vi "excelrowconcat_singlecol_LR_HR.vi"() -> ()   [LabVIEW 2020]
uses:
  <vilib>/addons/_office/excel.llb/Excel Get Data ([dbl]).vi
  <vilib>/Utility/file.llb/Write To Spreadsheet File (DBL).vi
  <vilib>/Utility/NIReport.llb/NI_report.lvclass
  <vilib>/Utility/NIReport.llb/Excel/NI_Excel.lvclass
  <vilib>/addons/_office/NI_ReportGenerationToolkit.lvlib
panel:
  out "Total LR Selected Row":i32=3
  in  "Tab Control":enum32{"HR", "LR"}(tab)=enum."LR"
  out "HR selected row":ext[](array[numeric])=[5.0, 20.0, 35.0, 50.0] format="%#_6f"
  out "HR Sheet Values":ext[][](array[numeric])=[[1.0, 16.0, 31.0, 46.0], [2.0, 17.0, 32.0, 47.0], [3.0, 18.0, 33.0, 48.0], [4.0, 19.0, 34.0, 49.0], [5.0, 20.0, 35.0, 50.0], [6.0, 21.0, 36.0, 51.0], [7.0, 22.0, 37.0, 52.0], [8.0, 23.0, 38.0, 53.0], [9.0, 24.0, 39.0, 54.0], [10.0, 25.0, 40.0, 55.0], [11.0, 26.0, 41.0, 56.0], [12.0, 27.0, 42.0, 57.0], [13.0, 28.0, 43.0, 58.0], [14.0, 29.0, 44.0, 59.0], [15.0, 30.0, 45.0, 60.0]] format="%_6f"
  out "HR Added row":ext[][](array[numeric])=[[1.0, 16.0, 31.0, 46.0], [3.0, 18.0, 33.0, 48.0], [5.0, 20.0, 35.0, 50.0]] format="%#_6f"
  out "HR Selected Column":ext[](array[numeric])=[46.0, 48.0, 50.0] format="%#_6f"
  out "HR Stack Col":ext[](array[numeric])=[1.0, 3.0, 5.0, 16.0, 18.0, 20.0, 31.0, 33.0, 35.0, 46.0, 48.0, 50.0] format="%#_6f"
  out "Rows":i32=15
  out "Columns":i32=4
  out "LR selected row":ext[](array[numeric])=[6.0, 21.0, 36.0, 51.0] format="%#_6f"
  out "LR Sheet Values":ext[][](array[numeric])=[[1.0, 16.0, 31.0, 46.0], [2.0, 17.0, 32.0, 47.0], [3.0, 18.0, 33.0, 48.0], [4.0, 19.0, 34.0, 49.0], [5.0, 20.0, 35.0, 50.0], [6.0, 21.0, 36.0, 51.0], [7.0, 22.0, 37.0, 52.0], [8.0, 23.0, 38.0, 53.0], [9.0, 24.0, 39.0, 54.0], [10.0, 25.0, 40.0, 55.0], [11.0, 26.0, 41.0, 56.0], [12.0, 27.0, 42.0, 57.0], [13.0, 28.0, 43.0, 58.0], [14.0, 29.0, 44.0, 59.0], [15.0, 30.0, 45.0, 60.0]] format="%_6f"
  out "LR Added row":ext[][](array[numeric])=[[2.0, 17.0, 32.0, 47.0], [4.0, 19.0, 34.0, 49.0], [6.0, 21.0, 36.0, 51.0]] format="%#_6f"
  out "LR Selected Column":ext[](array[numeric])=[47.0, 49.0, 51.0] format="%#_6f"
  out "LR Stack Col":ext[](array[numeric])=[2.0, 4.0, 6.0, 17.0, 19.0, 21.0, 32.0, 34.0, 36.0, 47.0, 49.0, 51.0] format="%#_6f"
  in  "LR state  Row Number (2,4,)":string="2,4,6"
  in  "Excel._Worksheet":refnum<k7>
  in  "Excel._Application":refnum<k7>
  in  "precission":string="6"
  in  "Destination path for cutting rows":path=path "C:/Users/lab user/Desktop/cm/single column"
  in  "row cut file name (no extension)":string="SCDUAL"
  in  "HR state  Row Number (1,3,)":string="1,3,5"
  out "Total HR Selected Row":i32=3
  in  "Select Excel file":path=path "C:/Users/lab user/Desktop/cm/single column/sc.xls"
  # "HR column stack output will be save in same directory\nrow cut file name_HR_single_col.xls"
  # "LR column stack output will be save in same directory\nrow cut file name_LR_single_col.xls"
  # "HR Row cut output will be save in same directory\nrow cut file name_HR.xls"
  # "LR Row cut  output will be save in same directory\nrow cut file name_LR.xls"
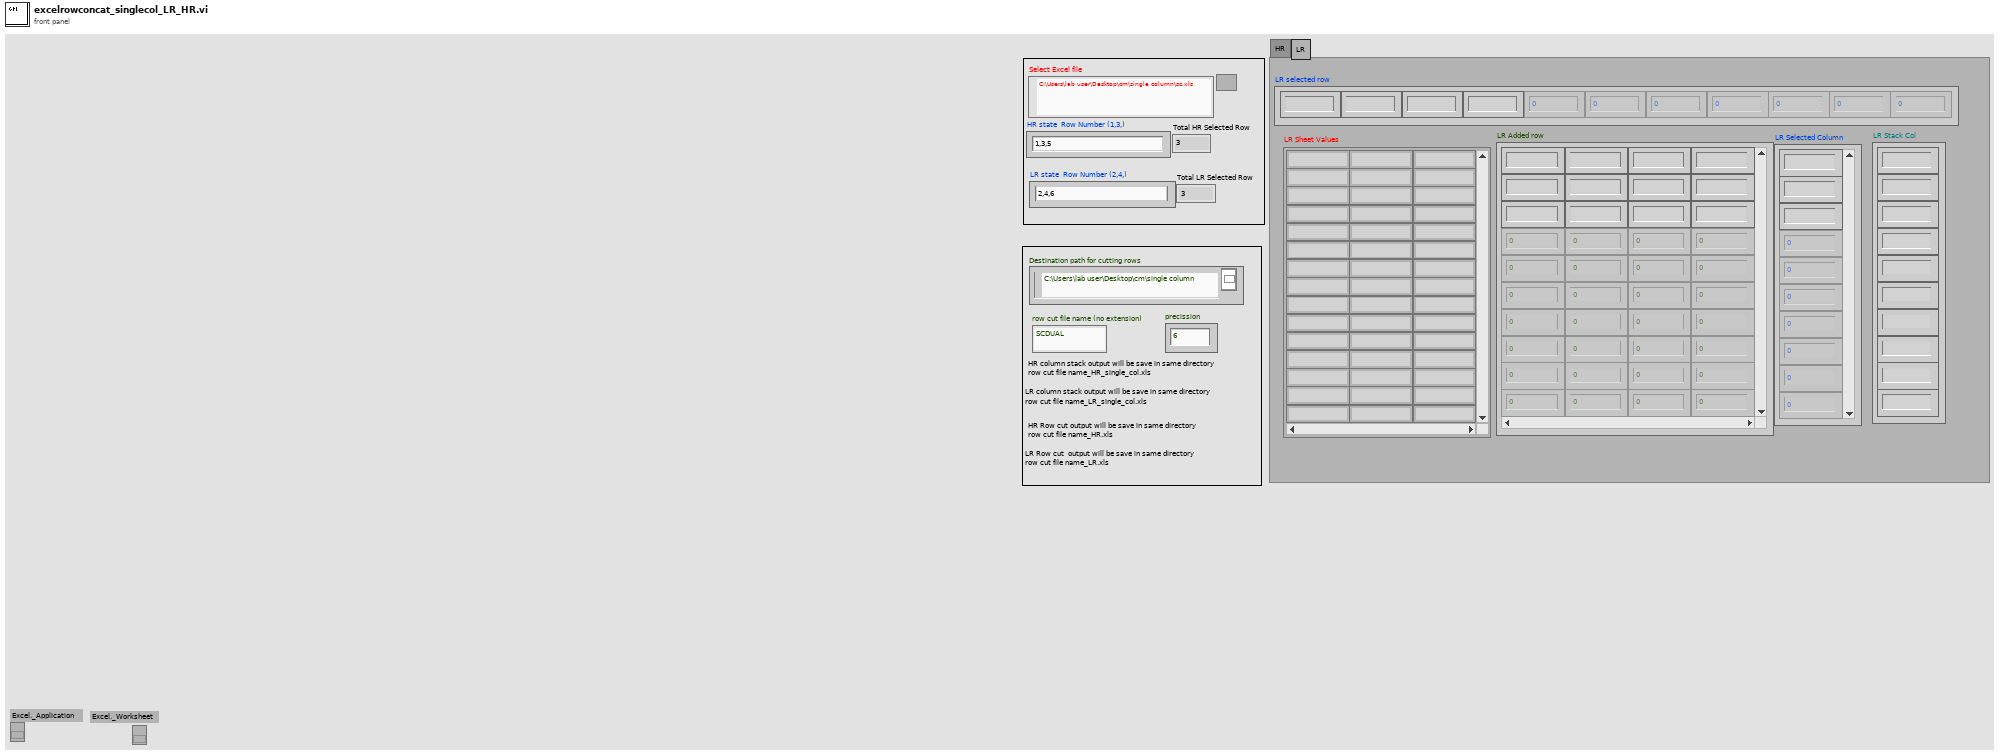
[diagram p1: front panel]
types:
  T1 = enum16{"Standard Report", "HTML", "Word", "Excel"}
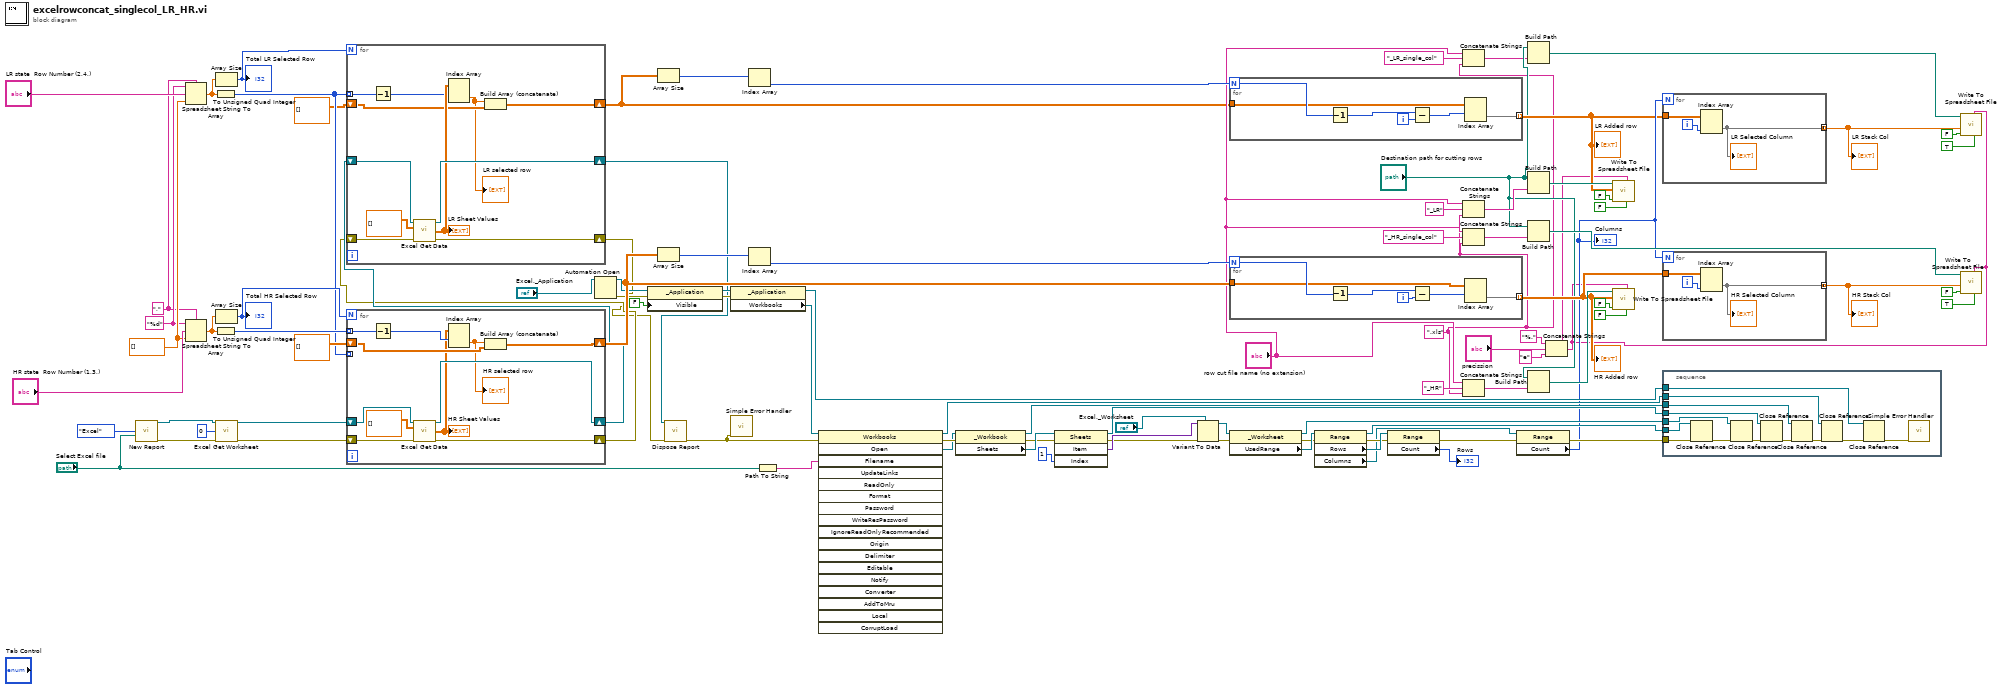
[diagram p0: block diagram]
diagram:
  w17 = ".xls" ("string")
  w36 = dbl[] []
  w33 = "," ("delimiter (Tab)")
  w34 = "%d" ("format string")
  n1 = call <vilib>:"New Report.vi"("report type"=T1."Excel", "template (empty)"="Select Excel file") -> ("report out"=w88:refnum<class "NI_report.lvclass">, "error out"=w89:errorcluster)  [unwired: 12 in]
  n2 = Spreadsheet String To Array(delimiter (Tab)=w33, format string=w34, spreadsheet string="LR state  Row Number (2,4,)", array type (2D Dbl)=w36) -> (array=w13:dbl[])
  n3 = Spreadsheet String To Array(delimiter (Tab)=w33, format string=w34, spreadsheet string="HR state  Row Number (1,3,)", array type (2D Dbl)=w36) -> (array=w92:dbl[])
  n4 = To Unsigned Quad Integer(1:w13) -> (0:w11:u64[])
  n5 = To Unsigned Quad Integer(1:w92) -> (0:w91:u64[])
  n6 = Array Size(array=w13) -> (size(s)=w8:i32)
  "Total LR Selected Row" <- w8
  n7 = Array Size(array=w92) -> (size(s)=w71:i32)
  "Total HR Selected Row" <- w71
  n8 = call <vilib>:"Excel Get Worksheet.vi"("report in"=w88, "worksheet index (0)"=0, "error in (no error)"=w89) -> ("report out"=w12:refnum<class "NI_report.lvclass">, "error out"=w87:errorcluster)  [unwired: 11 in]
  n9 = for {
    N: w71 -> [_]
    shift-right: [w105] -> w6
    shift-left: w12 -> [w100]
    shift-right: [w104] -> w5
    shift-left: w87 -> [w101]
    shift-right: [w102] -> w86
    shift-left: ext[][] [] -> [w103]
    tunnel: w91 -> [w99] mode=indexing
    tunnel: w11 -> [_] mode=indexing
    n10 = Decrement(x=w99) -> (x-1=w98:u64)
    n11 = call-poly <vilib>:"Excel Get Data.vi"("report in"=w100, "data type"=ext[][] [], "error in (no error)"=w101) -> ("report out"=w105:refnum<class "NI_report.lvclass">, "data"=w96:ext[][], "error out"=w104:errorcluster)  [unwired: 10 in]
    "HR Sheet Values" <- w96
    n12 = Index Array(array=w96, index (row)=w98) -> (element=w97:ext[])  [unwired: 1 in]
    "HR selected row" <- w97
    n13 = Build Array (concatenate)(w97, w103) -> (w102:ext[][])
  }
  n14 = for {
    N: w8 -> [_]
    shift-right: [w116] -> w4
    shift-left: w6 -> [w113]
    shift-right: [w115] -> w3
    shift-left: w5 -> [w114]
    tunnel: w11 -> [w111] mode=indexing
    shift-right: [w109] -> w10
    shift-left: ext[][] [] -> [w108]
    n15 = Decrement(x=w111) -> (x-1=w110:u64)
    n16 = call-poly <vilib>:"Excel Get Data.vi"("report in"=w113, "data type"=ext[][] [], "error in (no error)"=w114) -> ("report out"=w116:refnum<class "NI_report.lvclass">, "data"=w112:ext[][], "error out"=w115:errorcluster)  [unwired: 10 in]
    "LR Sheet Values" <- w112
    n17 = Index Array(array=w112, index (row)=w110) -> (element=w107:ext[])  [unwired: 1 in]
    "LR selected row" <- w107
    n18 = Build Array (concatenate)(w107, w108) -> (w109:ext[][])
  }
  n19 = Automation Open(Automation Refnum="Excel._Application") -> (Automation Refnum=w63:refnum<k7>, error out=w66:errorcluster)  [unwired: 3 in]
  n20 = property class="_Application"(reference=w63, error in=w66, "Visible"=FALSE ("Make Excel Visible")) -> (reference out=w62:refnum<k7>, error out=w65:errorcluster)
  n21 = Array Size(array=w10) -> (size(s)=w31:i32[])
  n22 = Array Size(array=w86) -> (size(s)=w84:i32[])
  n23 = call-dynamic "Dispose Report.vi"("report in"=w4, "error in (no error)"=w3) -> ("error out"=w39:errorcluster)  [unwired: 13 in]
  n24 = property class="_Application"(reference=w62, error in=w65) -> (reference out=w48:refnum<k7>, "Workbooks"=w51:refnum<k7>)  [unwired: 1 out]
  n25 = call <vilib>:"Simple Error Handler.vi"("error in (no error)"=w39) -> ()  [unwired: 4 in, 5 out]
  n26 = Index Array(array=w31) -> (element=w30:i32)  [unwired: 1 in]
  n27 = Index Array(array=w84) -> (element=w85:i32)  [unwired: 1 in]
  n28 = Path To String(path="Select Excel file") -> (string=w40:string)
  n29 = invoke class="Workbooks" method="Open"(reference=w51, error in=w39, "Filename"=w40) -> (reference out=w47:refnum<k7>, error out=w69:errorcluster, "Open"=w57:refnum<k7>)  [unwired: 15 in, 15 out]
  n30 = property class="_Workbook"(reference=w57, error in=w69) -> (reference out=w46:refnum<k7>, error out=w56:errorcluster, "Sheets"=w58:refnum<k7>)
  n31 = invoke class="Sheets" method="Item"(reference=w58, error in=w56, "Index"=1) -> (reference out=w45:refnum<k7>, error out=w55:errorcluster, "Item"=w68:variant)  [unwired: 1 in, 1 out]
  n32 = Variant To Data(error in=w55, type="Excel._Worksheet", Variant=w68) -> (data=w59:refnum<k7>, error out=w54:errorcluster)
  n33 = for {
    N: w30 -> [w123]
    tunnel: w10 -> [w120]
    tunnel: [w118] -> w22 mode=indexing
    i -> [w121]
    n34 = Decrement(x=w123) -> (x-1=w122:i32)
    n35 = Subtract(x=w122, y=w121) -> (x-y=w119:i32)
    n36 = Index Array(array=w120, index (row)=w119) -> (element=w118:ext[])  [unwired: 1 in]
  }
  "LR Added row" <- w22
  n37 = for {
    N: w85 -> [w129]
    tunnel: w86 -> [w126]
    tunnel: [w124] -> w77 mode=indexing
    i -> [w127]
    n38 = Decrement(x=w129) -> (x-1=w128:i32)
    n39 = Subtract(x=w128, y=w127) -> (x-y=w125:i32)
    n40 = Index Array(array=w126, index (row)=w125) -> (element=w124:ext[])  [unwired: 1 in]
  }
  "HR Added row" <- w77
  n41 = property class="_Worksheet"(reference=w59, error in=w54) -> (reference out=w44:refnum<k7>, error out=w53:errorcluster, "UsedRange"=w60:refnum<k7>)
  n42 = property class="Range"(reference=w60, error in=w53) -> (reference out=w43:refnum<k7>, error out=w52:errorcluster, "Rows"=w61:refnum<k7>, "Columns"=w49:refnum<k7>)
  n43 = property class="Range"(reference=w61, error in=w52) -> (error out=w42:errorcluster, "Count"=→"Rows":i32)  [unwired: 1 out]
  n44 = Concatenate Strings("row cut file name (no extension)", "_LR_single_col" ("string"), w17) -> (w15:string)
  n45 = Concatenate Strings("row cut file name (no extension)", "_LR" ("string"), w17) -> (w24:string)
  n46 = Concatenate Strings("row cut file name (no extension)", "_HR_single_col" ("string"), w17) -> (w72:string)
  n47 = Concatenate Strings("row cut file name (no extension)", "_HR" ("string"), w17) -> (w37:string)
  n48 = property class="Range"(reference=w49, error in=w42) -> (error out=w41:errorcluster, "Count"=w29:i32)  [unwired: 1 out]
  "Columns" <- w29
  n49 = Build Path(base path="Destination path for cutting rows", name or relative path=w15) -> (appended path=w14:path)
  n50 = Build Path(base path="Destination path for cutting rows", name or relative path=w24) -> (appended path=w23:path)
  n51 = Build Path(base path="Destination path for cutting rows", name or relative path=w72) -> (appended path=w74:path)
  n52 = Build Path(base path="Destination path for cutting rows", name or relative path=w37) -> (appended path=w81:path)
  n53 = Concatenate Strings("%.", "precission", "e") -> (w7:string)
  n54 = call-poly <vilib>:"Write To Spreadsheet File.vi"("transpose? (no:F)"=FALSE, "format (%.3f)"=w7, "append to file? (new file:F)"=FALSE, "2D data"=w22, "file path (dialog if empty)"=w23) -> ()  [unwired: 3 in, 1 out]
  n55 = call-poly <vilib>:"Write To Spreadsheet File.vi"("transpose? (no:F)"=FALSE, "format (%.3f)"=w7, "append to file? (new file:F)"=FALSE, "2D data"=w77, "file path (dialog if empty)"=w81) -> ()  [unwired: 3 in, 1 out]
  n56 = for {
    N: w29 -> [_]
    tunnel: w22 -> [w131]
    tunnel: [w130] -> w2 mode=concatenating
    i -> [w132]
    n57 = Index Array(array=w131, index (col)=w132) -> (element=w130:ext[])  [unwired: 1 in]
    "LR Selected Column" <- w130
  }
  "LR Stack Col" <- w2
  n58 = for {
    N: w29 -> [_]
    tunnel: w77 -> [w134]
    tunnel: [w133] -> w1 mode=concatenating
    i -> [w135]
    n59 = Index Array(array=w134, index (col)=w135) -> (element=w133:ext[])  [unwired: 1 in]
    "HR Selected Column" <- w133
  }
  "HR Stack Col" <- w1
  n60 = stacked-sequence {
    tunnel: w48 -> [w148]
    tunnel: w47 -> [w147]
    tunnel: w46 -> [w146]
    tunnel: w45 -> [w145]
    tunnel: w44 -> [w144]
    tunnel: w43 -> [w143]
    tunnel: w41 -> [w142]
    frame #0 {
      n61 = Close Reference(reference=w143, error in (no error)=w142) -> (error out=w141:errorcluster)
      n62 = Close Reference(reference=w144, error in (no error)=w141) -> (error out=w140:errorcluster)
      n63 = Close Reference(reference=w145, error in (no error)=w140) -> (error out=w139:errorcluster)
      n64 = Close Reference(reference=w146, error in (no error)=w139) -> (error out=w138:errorcluster)
      n65 = Close Reference(reference=w147, error in (no error)=w138) -> (error out=w137:errorcluster)
      n66 = Close Reference(reference=w148, error in (no error)=w137) -> (error out=w136:errorcluster)
      n67 = call <vilib>:"Simple Error Handler.vi"("error in (no error)"=w136) -> ()  [unwired: 4 in, 5 out]
    }
  }
  n68 = call-poly <vilib>:"Write To Spreadsheet File.vi"("transpose? (no:F)"=TRUE, "format (%.3f)"=w7, "append to file? (new file:F)"=FALSE, "1D data"=w2, "file path (dialog if empty)"=w14) -> ()  [unwired: 3 in, 1 out]
  n69 = call-poly <vilib>:"Write To Spreadsheet File.vi"("transpose? (no:F)"=TRUE, "format (%.3f)"=w7, "append to file? (new file:F)"=FALSE, "1D data"=w1, "file path (dialog if empty)"=w74) -> ()  [unwired: 3 in, 1 out]
